vi "llenaTablaTemporal.vi"(0 "Tbl Refnum":refnum<vi>, 1 "New Value":string[][](array[string]), 3 "error out":errorcluster) -> (7 "max value":dbl, 10 "error in (no error)":errorcluster)   [LabVIEW 2019, in "Prueba08.lvclass"]
uses:
  Prueba08.lvclass
  Prueba/Prueba.lvclass
panel:
  out "tablaTemp(num)":dbl[](array[numeric])
  out "output array":string[](array[string])
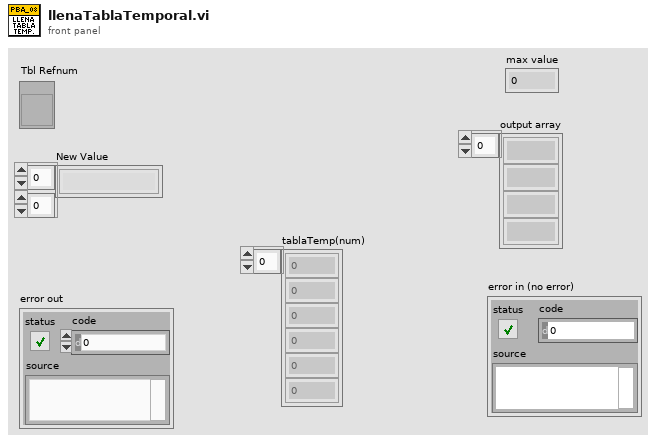
[diagram p1: front panel]
types:
  T1 = typedef "LVRowAndColumnTypeDef.ctl" = cluster{"Row":i32, "Column":i32}
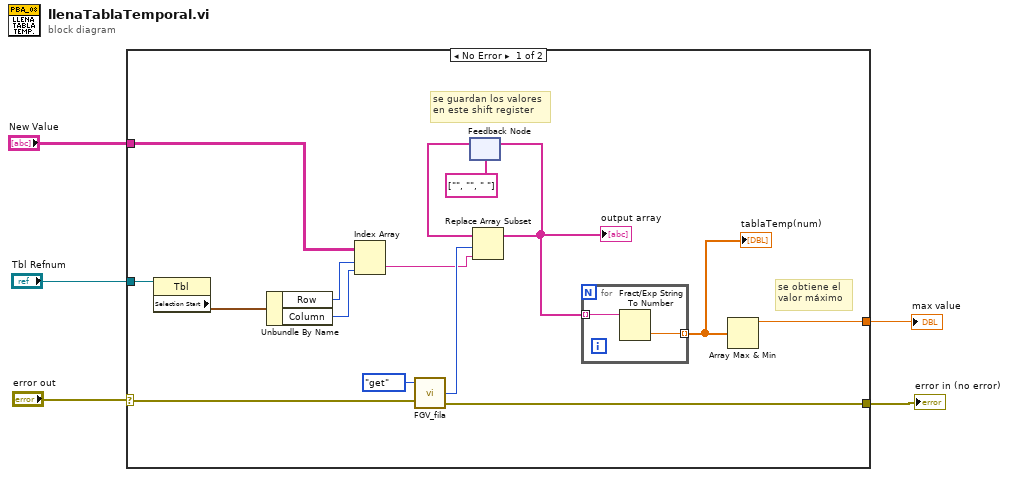
[diagram p0: block diagram]
diagram:
  n1 = case shown="No Error" "error out" {
    selector: "error out" -> [w8 w23]
    tunnel: "Tbl Refnum" -> [w12 _]
    tunnel: "New Value" -> [w11 _]
    tunnel: [w10 _] -> w3
    tunnel: [w7 w23] -> w1
    frame No Error {
      # "se obtiene el\nvalor máximo"
      # "se guardan los valores\nen este shift register"
      n2 = property on="Property Node" class="Tbl"(reference=w12) -> ("Selection Start"=w20:T1)  [unwired: 1 in, 2 out]
      n3 = Unbundle By Name(w20) -> ("Row"=w19:i32, "Column"=w18:i32)
      n4 = Index Array(array=w11, index (row)=w19, index (col)=w18) -> (element=w13:string)
      n5 = call "FGV_fila.vi"("error in (no error)"=w8, "action"=enum16{"increment", "set_start", "get"}."get") -> ("error out"=w7:errorcluster, "fila out"=w15:i32)  [unwired: 2 in]
      n6 = feedback #1(string[] ["", "", " "] ("NewVal")) -> (w16:string[])
      n7 = Replace Array Subset(array=w16, new element=w13, index=w15) -> (w6:string[])
      "output array" <- w6
      n8 = feedback-in #1(w6) -> ()
      n9 = for {
        tunnel: [w22] -> w9 mode=indexing
        tunnel: w6 -> [w21] mode=indexing
        n10 = Fract/Exp String To Number(string=w21) -> (number=w22:dbl)  [unwired: 3 in, 1 out]
      }
      "tablaTemp(num)" <- w9
      n11 = Array Max & Min(array=w9) -> (max value=w10:dbl)  [unwired: 3 out]
    }
    frame Error {
    }
  }
  "max value" <- w3
  "error in (no error)" <- w1
